vi "Soft_Robot_Model3.vi"() -> ()   [LabVIEW 2015]
uses:
  <vilib>/rvi/interface/nirviReadWriteControl/nirviReadWriteControl.xnode
  <vilib>/Utility/error.llb/Error Cluster From Error Code.vi
  <vilib>/rvi/errors/niLvFpgaAdjustHostInterfaceError.vi
  <vilib>/rvi/interface/nirviCloseFPGA/nirviCloseFPGA.xnode
  <vilib>/addons/Control Design/_Model Construction/NI_LinSys_Model Creation.lvlib
  <vilib>/Simulation/Implementation/XNodeFramework/SimXNode/SimX.xnode
  <vilib>/rvi/interface/nirviOpenFPGA/nirviOpenFPGA.xnode
  <vilib>/Platform/TimedLoop/XDataNode/XDataNode.xnode
  <vilib>/Platform/TimedLoop/XDataNode/nitl_modes.ctl
  <vilib>/Platform/TimedLoop/XDataNode/XDNodeRunTimeDep.lvlib
  <vilib>/Platform/TimedLoop/XDataNode/wakeup.ctl
  <vilib>/Platform/TimedLoop/XDataNode/timing_clust.ctl
  NiFpgaLv.dll
  <vilib>/rvi/interface/Simulation/niFpgaSimulationCallBeginRW.vi
  <vilib>/FPGAPlugInAG/Dynamic/niLvFpga_Close_Dynamic.vi
  <vilib>/addons/Control Design/_Implementation/CD State Feedback Controller.vi
  <vilib>/addons/Control Design/_Implementation/NI_CD_Implementation.lvlib
  <vilib>/addons/Control Design/_Model Construction/Model Creation.llb/Model Creation SubVI/cd_Create State Space Model.vi
  <vilib>/addons/Control Design/_Implementation/CD State Feedback Controller (Multiple Outputs).vi
  <vilib>/Simulation/Scripting/Companion Diagram/SimConfigNode/SimDog.xnode
  <vilib>/Simulation/Implementation/Shared/SIMSCR Execution Mode.ctl
  <vilib>/Simulation/Scripting/Companion Diagram/SimConfigNode/_simSolvers.ctl
  <vilib>/Simulation/Scripting/Companion Diagram/SimConfigNode/SimParams.ctl
  <vilib>/Simulation/Estimation/Implementation/NILVSim Discrete Kalman Filter.llb/SIM Disc KF Pred and Corr with Pred Gain with Checking Indirect Sim.vi
  <vilib>/addons/Control Design/_Implementation/CD Continuous Recursive Kalman Filter.vi
  <vilib>/addons/Control Design/_Stochastic Systems/NI_CD_Stochastic Systems.lvlib
  <vilib>/addons/Control Design/_Stochastic Systems/Stochastic Systems.llb/CD Construct Stochastic Model (Numeric).vi
  <vilib>/addons/Control Design/_Stochastic Systems/Stochastic Systems.llb/CD Construct Noise Model (Numeric).vi
  <vilib>/Simulation/Implementation/Shared/SIM Bundle Sim Info.vi
  <vilib>/Simulation/Implementation/Shared/SIM Unbundle Sim Info.vi
  <vilib>/Simulation/Implementation/Shared/NILVSim_FinalizeModel.vi
  <vilib>/Simulation/Implementation/Shared/NILVSim_GetModelError.vi
  <vilib>/Simulation/Implementation/Shared/NILVSim_Initialize.vi
  <vilib>/Simulation/Implementation/Shared/NILVSim_FinishedLate.vi
  <vilib>/Simulation/Utility/Implementation/NILVSim Get Time and IsAcceptedStep.vi
  <vilib>/Simulation/Implementation/Shared/NILVSim_Manager.vi
  <vilib>/Simulation/Implementation/Shared/NI_SIM_Implementation.lvlib
  <vilib>/Simulation/Implementation/Shared/NILVSIM_BeginStep.vi
  <vilib>/Simulation/Param Hierarchy/Typedefs/SIMPH Param Control Actions.ctl
  <vilib>/Simulation/Implementation/Shared/NILVSim_ParamChanged.vi
  <vilib>/Utility/error.llb/Clear Errors.vi
  <vilib>/Simulation/Implementation/Shared/SIMSH Read Queue.vi
  <vilib>/addons/Control Design/_Stochastic Systems/Stochastic Systems.llb/Stochastic Systems SubVIs/cd_Second-Order Statistics Noise Model.ctl
  FPGA Bitfiles/ACC20115_FPGATarget_CurrentControlle_Dt5vFgOzYtY.lvbitx
  Current Controller.vi
  <vilib>/FPGAPlugInAG/myRIO-1900/niLvFpga_Open_myRIO-1900.vi
  <vilib>/rvi/interface/common/dynamic/niFpgaDynamicAddResources.vi
  <vilib>/addons/Control Design/_Model Construction/Model Typedefs.llb/CD General Elements.ctl
  <vilib>/addons/Control Design/_Model Construction/NI_LinSys_Model Typedefs.lvlib
  <vilib>/addons/Control Design/_Model Construction/Model Typedefs.llb/CD State Space Model (MIMO).ctl
panel:
  in  "SP":dbl(slide) scale=0.0..100.0
  in  "Tab Control":enum32{"Outputs", "Inputs"}(tab)
  out "KF Post":dbl[](graph)
  out "DAC Inlet Valve 2":i32(graph)
  in  "Current (mA)":i32
  out "Status?":bool
  out "State-Space Model":T1={"properties"={"Model name"="", "Input names"=[], "Output names"=[], "Input Delays"=[], "Output Delays"=[], "Sampling Time"=0.0, "Notes"=""}, "A"=[], "B"=[[3.03e-07], [4.04e-07]], "C"=[], "D"=[], "StateNames"=[], "Transport Delay"=[]} {"Transport Delay" format="%.2f"; "D" format="%#.2g"; "C" format="%#.2g"; "B" format="%#.2g"; "A" format="%#.2g"; "properties"."Sampling Time" format="%#.6p"; "properties"."Output Delays" format="%.4f"; "properties"."Input Delays" format="%.4f"}
  out "KF Gain M(k)":dbl[][](array[numeric])
  out "Fusion Data":dbl(graph)
  in  "Stop":bool
  out "xhat(t)":dbl[](array[numeric])
  in  "A":dbl[][](array[numeric])=[[1.01, -0.1716], [0.001556, 0.9782]] format="%#.5g"
  in  "B":dbl[][](array[numeric]) format="%#.5g"
  in  "C":dbl[][](array[numeric])=[[1.089, -0.03769]] format="%#.5g"
  out "error out":errorcluster
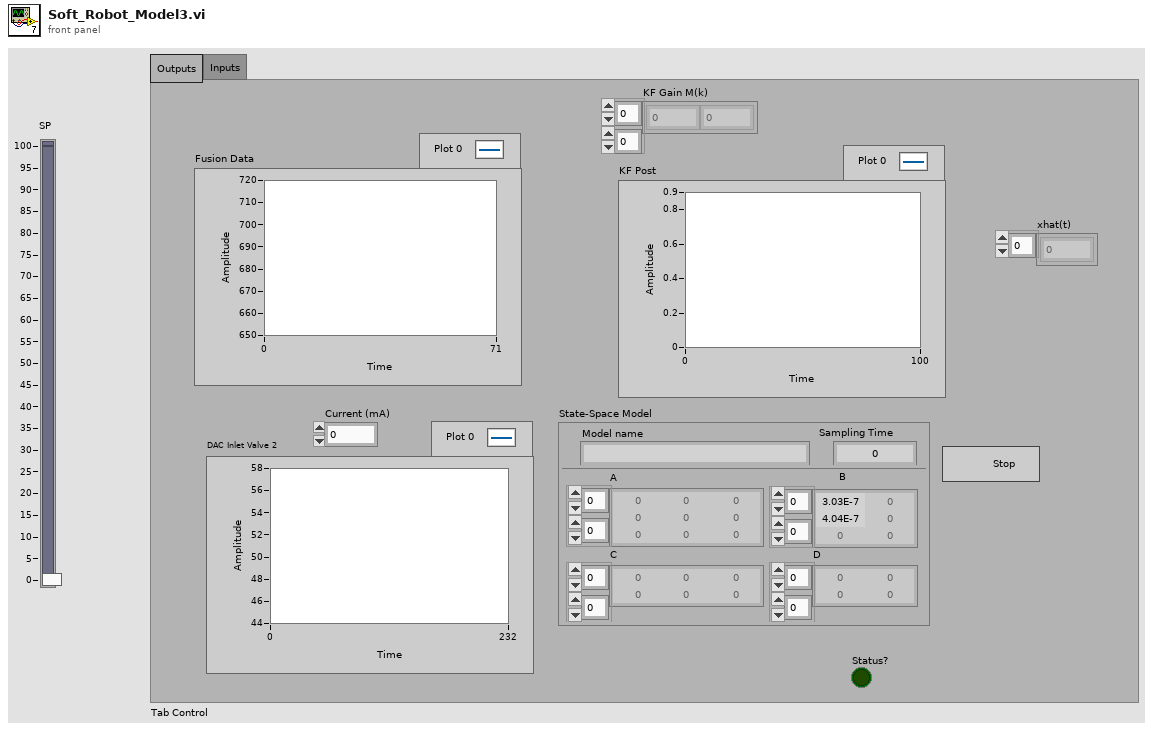
[diagram p1: front panel]
types:
  T1 = typedef "NI_LinSys_Model Typedefs.lvlib/CD State Space Model (MIMO).ctl" = cluster{"properties":T2, "A":dbl[][], "B":dbl[][], "C":dbl[][], "D":dbl[][], "StateNames":string[], "Transport Delay":dbl[][]}
  T2 = typedef "NI_LinSys_Model Typedefs.lvlib/CD General Elements.ctl" = cluster{"Model name":string, "Input names":string[], "Output names":string[], "Input Delays":dbl[], "Output Delays":dbl[], "Sampling Time":dbl, "Notes":string}
  T3 = typedef "XDNodeRunTimeDep.lvlib/timing_clust.ctl" = cluster{"Expected End [f-1]":u64, "Actual End [f-1]":u64, "Finished Late? [f-1]":bool, "Expected End [i-1]":u64, "Actual End [i-1]":u64, "Finished Late? [i-1]":bool, "Expected Start [i]":u64, "Actual Start [i]":u64, "Expected Start [f]":u64, "Actual Start [f]":u64, "Source Name":string, "Structure Name":string, "Period":i64, "Deadline":i64, "Offset":i64, "Start":i64, "Priority":i32, "Timeout":i32, "Mode":T4, "Wakeup Reason":T5, "Error":errorcluster, "Source Type":string, "Secondary Source Type":string, "Global End Time":u64, "Global Start Time":u64, "Frame Duration":u64, "Iteration Duration":u64, "Assigned CPU":i32, "I/O Scan Engine Mode":u32}
  T4 = typedef "XDNodeRunTimeDep.lvlib/nitl_modes.ctl" = enum32{"No Change", "Process missed periods, maintain original phase", "Discard missed periods, maintain original phase", "Process missed periods, ignore original phase", "Discard missed periods, ignore original phase"}
  T5 = typedef "XDNodeRunTimeDep.lvlib/wakeup.ctl" = enum32{"Normal", "Aborted", "Asynchronous wakeup", "Timing source error", "Timed loop error", "Timeout"}
  T6 = typedef "NI_CD_Stochastic Systems.lvlib/cd_Stochastic State-Space Model.ctl" = cluster{"Sampling Time (s)":dbl, "G":dbl[][], "B":dbl[][], "A":dbl[][], "C":dbl[][], "D":dbl[][], "H":dbl[][]}
  T7 = typedef "NI_CD_Stochastic Systems.lvlib/cd_Second-Order Statistics Noise Model.ctl" = cluster{"Q":dbl[][], "E{w}":dbl[], "E{v}":dbl[], "R":dbl[][], "N":dbl[][]}
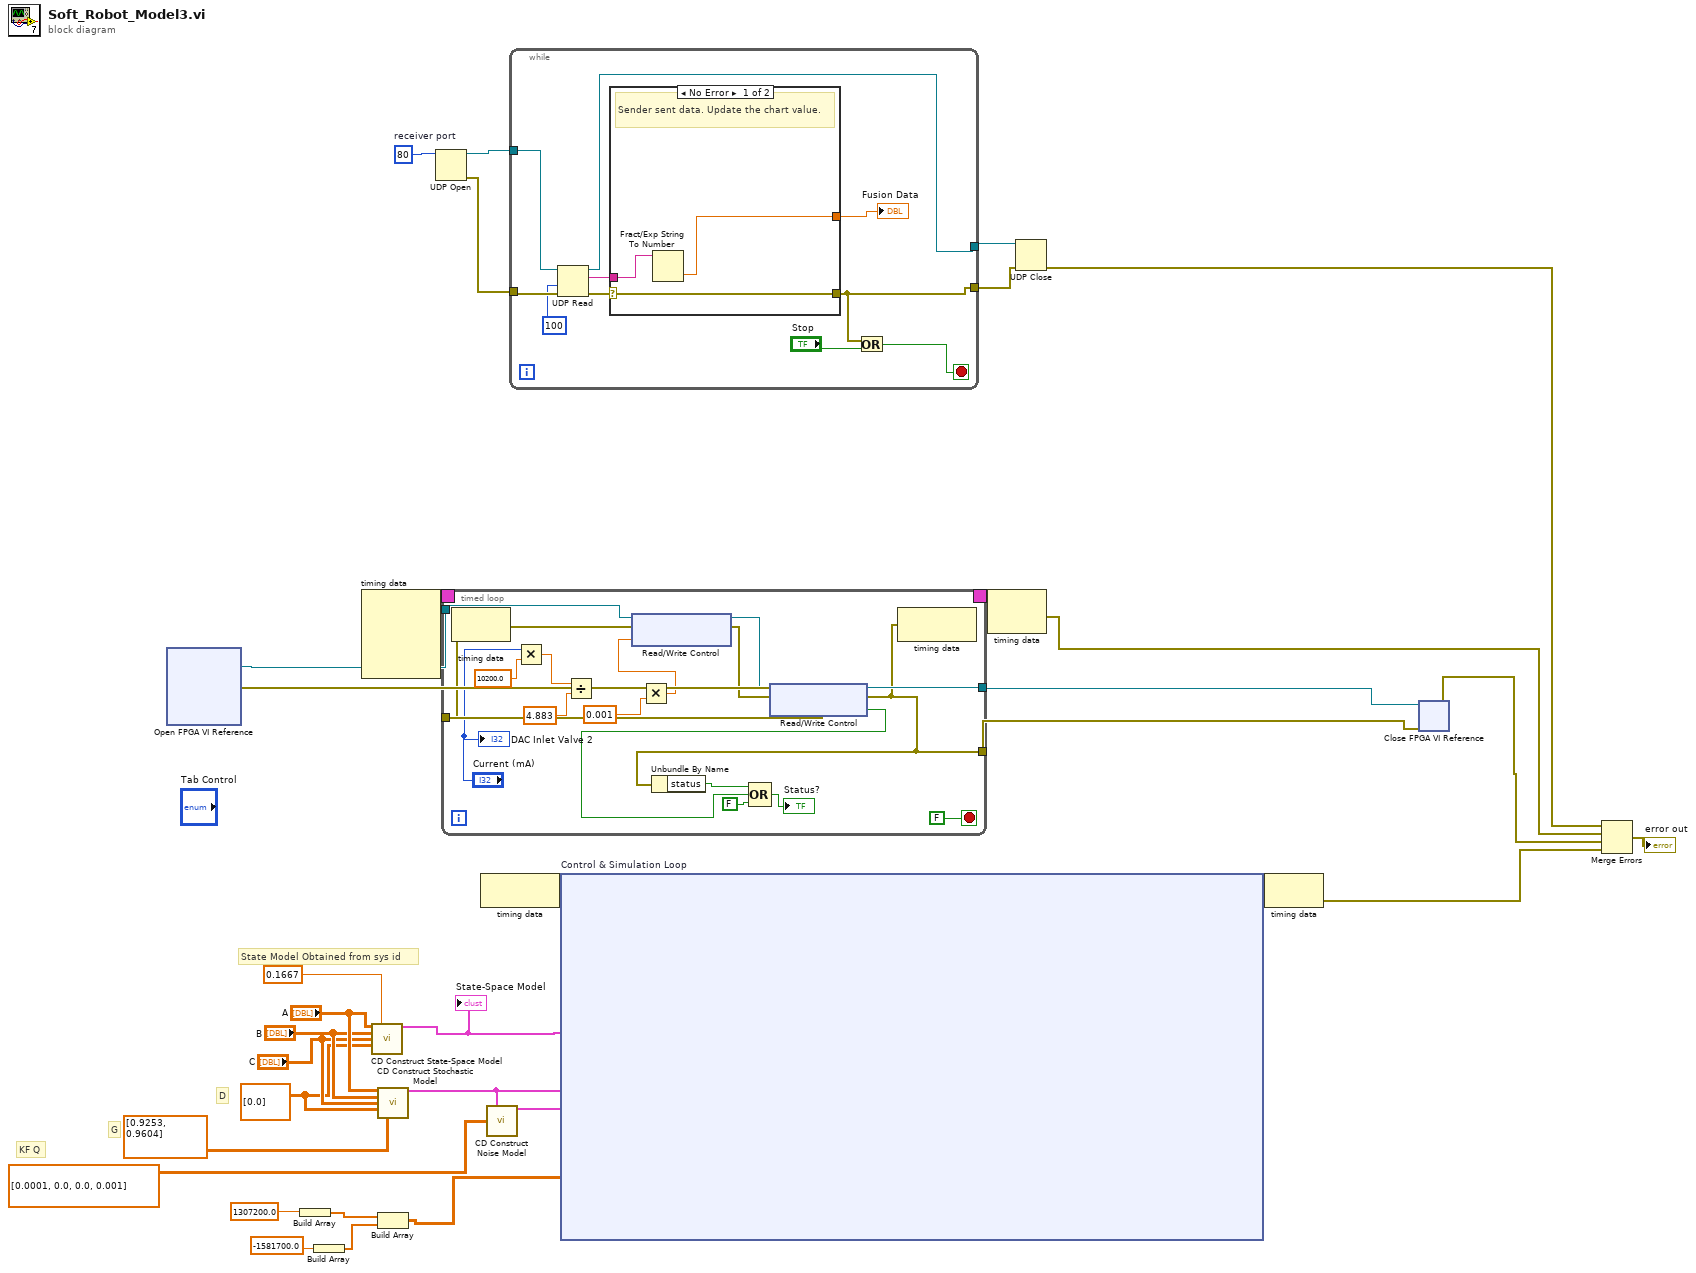
[diagram p0: block diagram]
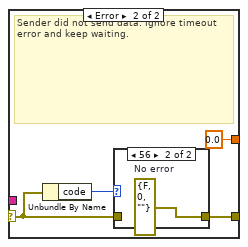
[diagram p2: hidden frame]
diagram:
  w6 = dbl[][] [[0.0]] ("D")
  w18 = u16 80  # receiver port
  # "KF Q"
  # "D"
  # "G"
  # "State Model Obtained from sys id"
  n1 = xnode "Open FPGA VI Reference"() -> ("FPGA VI Reference Out"=w31:refnum<k20>, "error out"=w30:errorcluster)  [unwired: 2 in]
  n2 = Build Array(1307200.0 ("element")) -> (w21:dbl[])
  n3 = Build Array(-1581700.0 ("element")) -> (w20:dbl[])
  n4 = node-c288() -> (w29:T3)  [unwired: 4 in]
  n5 = call-poly <vilib>:"CD Construct State-Space Model.vi"("A"="A", "Sampling Time (s)"=0.1667, "B"="B", "C"="C", "D"=w6) -> ("State-Space Model"=w10:T1)  [unwired: 9 in, 1 out]
  "State-Space Model" <- w10
  n6 = call-poly <vilib>:"CD Construct Stochastic Model.vi"("A"="A", "B"="B", "C"="C", "D"=w6, "G"=dbl[][] [[0.9253], [0.9604]]) -> ("Stochastic State-Space Model"=w4:T6)  [unwired: 9 in, 1 out]
  n7 = Build Array(w21, w20) -> (w19:dbl[][])
  n8 = UDP Open(11:w18) -> (port=w17:refnum<k16>, 0:w16:errorcluster)  [unwired: 4 in, 1 out]
  n9 = timed-loop {
    tunnel: w31 -> [w50]
    tunnel: w30 -> [w35]
    tunnel: [w34] -> w26
    tunnel: [w43] -> w33
    timing: w29 -> [_]
    timing-out: [_] -> w28
    stop <- FALSE stop-if-true
    n10 = node-c288() -> ()  [unwired: 1 in, 1 out]
    n11 = Multiply(x="Current (mA)", y=10200.0) -> (x*y=w38:dbl)
    n12 = Divide(x=w38, y=4.883) -> (x/y=w41:dbl)
    n13 = Multiply(x=w41, y=0.001) -> (x*y=w37:dbl)
    n14 = xnode "Read/Write Control"("FPGA VI Reference In"=w50, "error in"=w35, "DAC Inlet Valve"=w37) -> ("FPGA VI Reference Out"=w49:refnum<k20>, "error out"=w48:errorcluster)
    n15 = xnode "Read/Write Control"("FPGA VI Reference In"=w49, "error in"=w48) -> ("FPGA VI Reference Out"=w43:refnum<k20>, "error out"=w34:errorcluster, "Inlet Overflow?"=w44:bool)
    n16 = Unbundle By Name(w34) -> ("status"=w46:bool)
    n17 = Compound Arithmetic op=OR(w46, w44, FALSE ("value")) -> (→"Status?":bool)
    n18 = node-c288(w34) -> ()  [unwired: 1 out]
    "DAC Inlet Valve 2" <- "Current (mA)"
  }
  n19 = node-c288() -> (w12:variant)  [unwired: 1 in]
  n20 = call-poly <vilib>:"CD Construct Noise Model.vi"("Stochastic State-Space Model"=w4, "Q"=dbl[][] [[0.0001, 0.0], [0.0, 0.001]]) -> ("Second-Order Statistics Noise Model out"=w2:T7)  [unwired: 12 in, 1 out]
  n21 = while {
    tunnel: w17 -> [w65]
    tunnel: w16 -> [w64]
    tunnel: [w58] -> w15
    tunnel: [w56] -> w14
    stop <- w57 stop-if-true
    n22 = UDP Read(connection ID=w65, timeout ms (25000)=100, 8:w64) -> (data out=w61:string, error out=w60:errorcluster, 3:w58:refnum<k16>)  [unwired: 3 out]
    n23 = case shown="No Error" w60 {
      selector: w60 -> [w67 w71]
      tunnel: w61 -> [w68 _]
      tunnel: [w67 w70] -> w56
      tunnel: [w66 0.0] -> w59
      frame No Error {
        # "Sender sent data. Update the chart value."
        n24 = Fract/Exp String To Number(string=w68) -> (number=w66:dbl)  [unwired: 3 in, 1 out]
      }
      frame Error {
        # "Sender did not send data. Ignore timeout error and keep waiting."
        n25 = Unbundle By Name(w71) -> ("code"=w72:i32)
        n26 = case shown="56" w72 {
          tunnel: w71 -> [w73 _]
          tunnel: [w73 w74] -> w70
          frame Default {
          }
          frame 56 {
            w74 = errorcluster {"status"=FALSE, "code"=0, "source"=""}  # No error
          }
        }
      }
    }
    "Fusion Data" <- w59
    n27 = Or(x=w56, y="Stop") -> (x .or. y?=w57:bool)
  }
  n28 = node-c254 "Control & Simulation Loop"(w12, w19, w10, w4, w2) -> (w11:variant)
  n29 = node-c288(w28) -> (w24:errorcluster)
  n30 = UDP Close(connection ID=w15, 8:w14) -> (error out=w13:errorcluster)  [unwired: 1 out]
  n31 = node-c288(w11) -> (w1:errorcluster)
  n32 = xnode "Close FPGA VI Reference"("FPGA VI Reference In"=w33, "error in"=w26) -> ("error out"=w25:errorcluster)
  n33 = Merge Errors(w13, w24, w25, w1) -> (→"error out":errorcluster)
